vi "SetHighPoint.vi"(8 "error in (no error)":errorcluster, 10 "High Temperature":i32) -> (0 "error out":errorcluster, 2 "Return String":string)   [LabVIEW 2017, in "Thermal Shock.lvlib"]
uses:
  Thermal Shock.lvlib
  <vilib>/Instr/_visa.llb/VISA Configure Serial Port (Instr).vi
panel:
  in  "Write Data!":bool=TRUE
  in  "Stop!":bool=TRUE
  out "VISA Resource Out":refnum<visa-resource-name>
  in  "VISA Resource In":refnum<visa-resource-name>
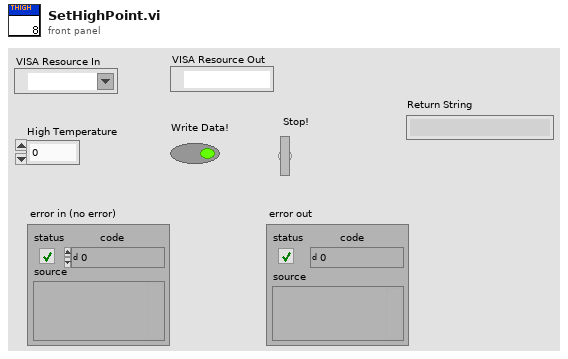
[diagram p1: front panel]
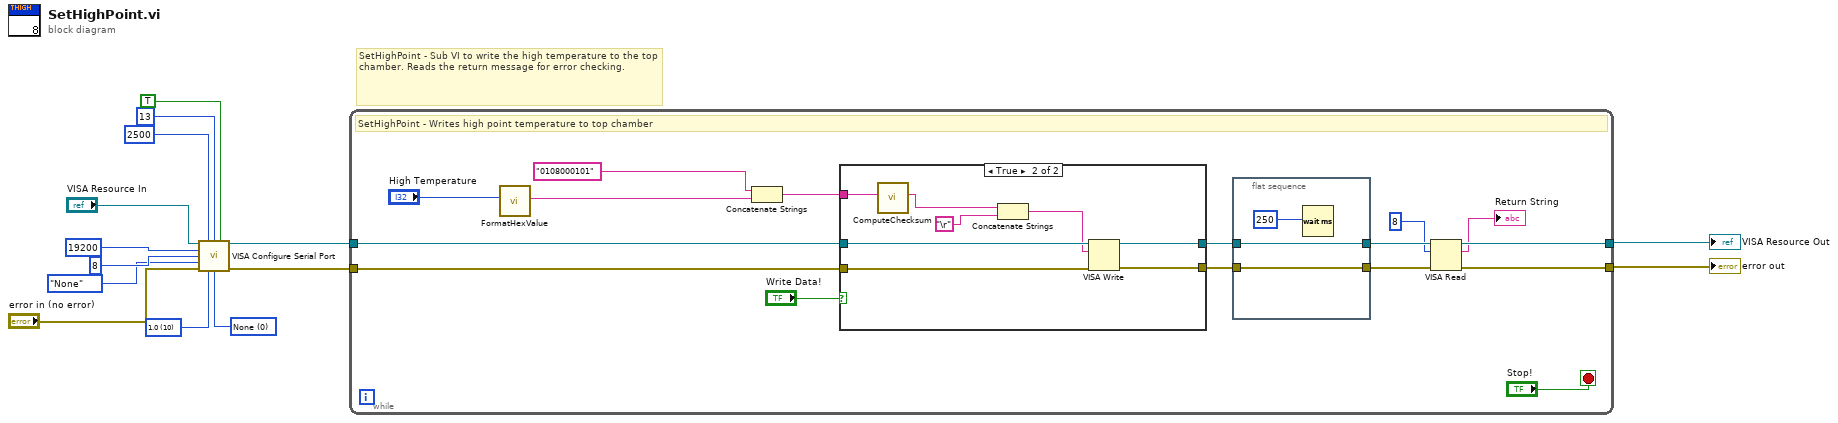
[diagram p0: block diagram]
diagram:
  w7 = u16 0 items=["None", "XON/XOFF", "RTS/CTS", "XON/XOFF & RTS/CTS", "DTR/DSR", "XON/XOFF & DTR/DSR"] ("flow control (0:none)")
  w9 = u16 10 items=["1.0"=10, "1.5"=15, "2.0"=20] ("stop bits (10: 1 bit)")
  # "SetHighPoint - Sub VI to write the high temperature to the top chamber. Reads the return message for error checking."
  n1 = call-poly "VISA Configure Serial Port"("VISA resource name"="VISA Resource In", "timeout (10sec)"=2500, "termination char\n(0xA = '\\n' = LF)"=u8 13, "Enable Termination\nChar (T)"=TRUE, "baud rate (9600)"=19200, "data bits (8)"=u16 8, "parity (0:none)"=enum16{"None", "Odd", "Even", "Mark", "Space"}."None", "error in (no error)"="error in (no error)", "stop bits (10: 1 bit)"=w9, "flow control (0:none)"=w7) -> ("VISA resource name out"=w4:refnum<visa-resource-name>, "error out"=w3:errorcluster)  [unwired: 4 in]
  n2 = while {
    tunnel: w4 -> [w29]
    tunnel: w3 -> [w28]
    tunnel: [w20] -> w2
    tunnel: [w19] -> w1
    stop <- "Stop!" stop-if-true
    # "SetHighPoint - Writes high point temperature to top chamber"
    n3 = call "FormatHexValue.vi"("Value"="High Temperature") -> ("FormattedValue"=w15:string)  [unwired: 10 in]
    n4 = Concatenate Strings("0108000101", w15) -> (w26:string)
    n5 = case shown="True" "Write Data!" {
      tunnel: w26 -> [_ w43]
      tunnel: w29 -> [w35 w42]
      tunnel: w28 -> [w34 w41]
      tunnel: [w35 w40] -> w24
      tunnel: [w34 w39] -> w23
      frame False {
      }
      frame True {
        n6 = call "ComputeChecksum.vi"("Input Command"=w43) -> ("Command Message"=w38:string)  [unwired: 9 in, 1 out]
        n7 = Concatenate Strings(w38, "\r") -> (w36:string)
        n8 = VISA Write(VISA resource name=w42, write buffer=w36, error in (no error)=w41) -> (VISA resource name out=w40:refnum<visa-resource-name>, error out=w39:errorcluster)  [unwired: 1 out]
      }
    }
    n9 = flat-sequence {
      tunnel: w24 -> [w32]
      tunnel: w23 -> [w31]
      tunnel: [w32] -> w22
      tunnel: [w31] -> w21
      frame #0 {
        n10 = Wait (ms)(milliseconds to wait=250) -> ()  [unwired: 1 out]
      }
    }
    n11 = VISA Read(VISA resource name=w22, byte count=8, error in (no error)=w21) -> (VISA resource name out=w20:refnum<visa-resource-name>, read buffer=→"Return String":string, error out=w19:errorcluster)  [unwired: 1 out]
  }
  "VISA Resource Out" <- w2
  "error out" <- w1
